vi "myRIO_BRig_RT_dataExp_nBlock.vi"() -> (2 "output_nBlock":i32)   [LabVIEW 2014]
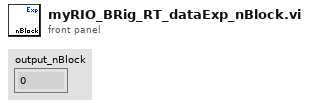
[diagram p1: front panel]
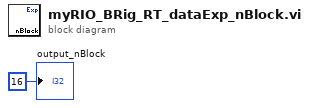
[diagram p0: block diagram]
diagram:
  "output_nBlock" <- 16 ("output_iBlock")
